vi "tcs shm issue Command start LV.vi"(8 "error in (no error)":errorcluster, 11 "command_start_Ctl":cluster{"size":i32, "data":string}) -> (0 "error out":errorcluster, 2 "function return":i32, 3 "command_start_Ctl out":cluster{"size":i32, "data":string})   [LabVIEW 2016, in "SALLV_tcs.lvlib"]
doc: "int tcs_shm_issueCommand_startLV(tcs_command_startLV *command_start_Ctl );"
uses:
  SALLV_tcs.lvlib
  SALLV_tcs.so
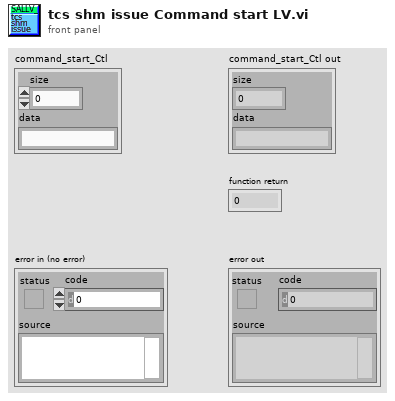
[diagram p1: front panel]
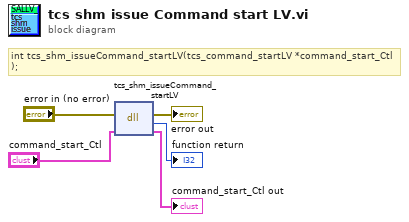
[diagram p0: block diagram]
diagram:
  # "int tcs_shm_issueCommand_startLV(tcs_command_startLV *command_start_Ctl );"
  n1 = dll-call lib="home/plotz/SALLV_tcs/SALLV_tcs.*" fn="tcs_shm_issueCommand_startLV"(error in="error in (no error)", "command_start_Ctl"="command_start_Ctl") -> (error out=→"error out":errorcluster, →"function return":i32, "command_start_Ctl"=→"command_start_Ctl out":cluster{"size":i32, "data":string})  [unwired: 2 in, 1 out]
